vi "Initialize.vi"(7 "not in use":string="Setpoint.ch%d.SP", 8 "error in":errorcluster, 9 "Number of Channels":u32=1, 10 "Instance Name":string="PluginName", 11 "Current Setpoint in":refnum<class "Current Setpoint.lvclass">) -> (0 "error out":errorcluster, 3 "Current Setpoint out":refnum<class "Current Setpoint.lvclass">)   [LabVIEW 2023, in "Current Setpoint.lvclass"]
uses:
  Current Setpoint.lvclass
  Parents/Setpoint/Setpoint.lvclass
  Current Setpoint.lvclass/Current Setpoint.ctl
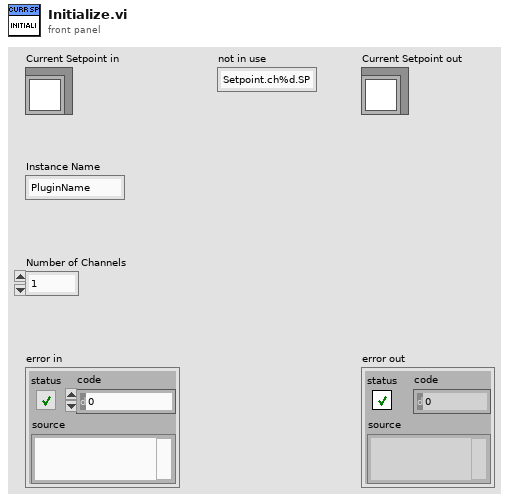
[diagram p1: front panel]
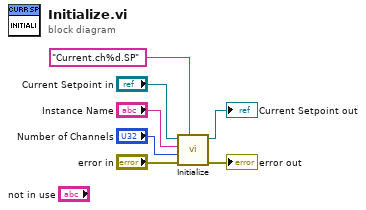
[diagram p0: block diagram]
diagram:
  n1 = call-parent "Initialize.vi"("ChannelName"="Current.ch%d.SP", "error in"="error in", "Number of Channels"="Number of Channels", "Instance Name"="Instance Name", "Setpoint in"="Current Setpoint in") -> ("error out"=→"error out":errorcluster, "Setpoint out"=→"Current Setpoint out":refnum<class "Current Setpoint.lvclass">)  [unwired: 5 in]
